vi "Initialize.vi"(7 "Path":path, 8 "error in (no error)":errorcluster, 9 "Invoked from wizard":bool, 10 "Object":T2, 11 "AB_UI_Fmwrk_Build in":refnum<class "AB_UI_Frmwk_Build.lvclass">) -> (0 "error out":errorcluster, 1 "helpTopics out":string[](array[string]), 2 "pageTitles out":string[](array[string]), 3 "AB_UI_Fmwrk_Build out":refnum<class "AB_UI_Frmwk_Build.lvclass">, 4 "helpFile":string, 5 "pageMsgData":T1[](array[typedef]))   [LabVIEW 2020, in "AB_UI_Frmwk_Build.lvclass"]
uses:
  <vilib>/AppBuilder/AB_Classes/Build/UI/AB_UI_Frmwk_Build.lvclass
  <resource>/Framework/Providers/API/ItemRef.ctl
  <resource>/Framework/Providers/Builds/AppBuilder/AB_UI_Page_MessageData.ctl
  <resource>/Framework/Providers/Builds/AppBuilder/AB_UI_Framework_MsgToPage_Action.ctl
  <resource>/Framework/Providers/Builds/AppBuilder/SRdB/AB_SRdB_Action.ctl
  <vilib>/AppBuilder/AB_Classes/Build/AB_Build.lvclass
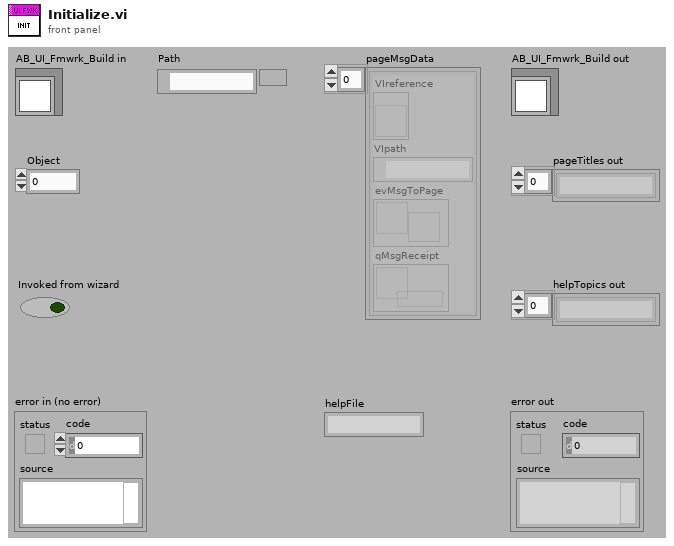
[diagram p1: front panel]
types:
  T1 = typedef "AB_UI_Page_MessageData.ctl" = cluster{"VIreference":refnum<vi>, "VIpath":path, "evMsgToPage":refnum<user-event>, "qMsgReceipt":refnum<queue>}
  T2 = typedef "ItemRef.ctl" = u64
  T3 = typedef "AB_SRdB_Action.ctl" = enum16{"read", "write", "create", "delete", "initialize", "unInitialize", "getLock", "readAll", "writeAll"}
  T4 = typedef "AB_Build.ctl" = cluster{"buildSpecName":string, "buildSpecDescription":string, "destinations":refnum<class "AB_Destination.lvclass">[], "exclusionOption":T5, "defaultLanguage":string, "supportedLanguages":string[], "excludedDirectories":path[], "buildContext":refnum<vi>, "buildObject":T2, "preview":bool, "programatic":bool, "progressBarEvents":T6, "userLog_Path":path, "preActionID":string, "preAction_Path":path, "postActionID":string, "postAction_Path":path, "eng_checkForBrokenVIs?":bool, "eng_verboseLinkerErrors?":bool, "localDest_Path":path, "targetDest_Path":path, "removeVIObject":u16, "cache":refnum<class "PreviewCache.lvclass">, "use cache":bool, "previewCache_ID":string, "buildCache_ID":string, "eng_TempLocalDest_Path":path, "eng_collectDependencies?":bool, "versionInfo":cluster{"buildVersion":cluster{"major":u16, "minor":u16, "patch":u16, "build":u16}, "autoIncrement":bool}, "eng_enableVIChecksums":bool}
  T5 = typedef "AB_Exclusion_Option.ctl" = cluster{"typedefs":bool, "polymorphicVIs":bool, "unusedLibraryItems":bool, "modifyLibraryFile":bool, "edit-timeDependencies":bool, "inlineVIs":bool, "dependent PPLs":bool, "dependent DLLs":bool}
  T6 = typedef "provcom_ProgressBar_Events.ctl" = cluster{"newJob":refnum<user-event>, "newItem":refnum<user-event>, "errorMsg":T7, "cancel":refnum<user-event>}
  T7 = typedef "mxLvBuildError.ctl" = refnum<user-event>
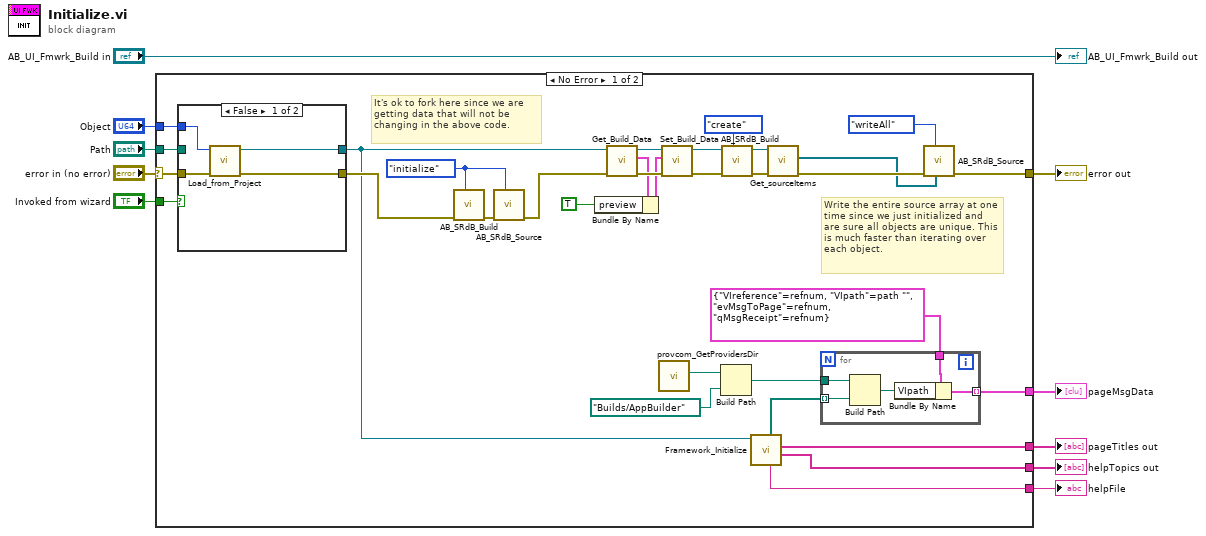
[diagram p0: block diagram]
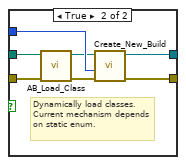
[diagram p2: hidden frame]
diagram:
  n1 = case shown="No Error" "error in (no error)" {
    selector: "error in (no error)" -> [w40 w59]
    tunnel: "Object" -> [w38 _]
    tunnel: [w12 w59] -> w4
    tunnel: [w39 _] -> w5
    tunnel: "Invoked from wizard" -> [w37 _]
    tunnel: [w18 _] -> w1
    tunnel: [w17 _] -> w3
    tunnel: [w19 _] -> w2
    tunnel: "Path" -> [w16 _]
    frame No Error {
      w33 = AB_SRdB_Action."initialize" ("action")
      # "Write the entire source array at one time since we just initialized and are sure all objects are unique. This is much faster than iterating over each object."
      # "It's ok to fork here since we are getting data that will not be changing in the above code."
      n2 = case shown="False" w37 {
        tunnel: [w43 w53] -> w35
        tunnel: w40 -> [w46 w50]
        tunnel: w38 -> [w45 w51]
        tunnel: [w44 w52] -> w21
        tunnel: w16 -> [_ w47]
        frame False {
          n3 = call <vilib>:"Load_from_Project.vi"("error in (no error)"=w46, "Object"=w45) -> ("error out"=w43:errorcluster, "Build out"=w44:refnum<class "AB_Build.lvclass">)  [unwired: 8 out]
        }
        frame True {
          # "Dynamically load classes. Current mechanism depends on static enum."
          n4 = call <vilib>:"AB_Load_Class.vi"("error in (no error)"=w50, "AB_Class path"=w47) -> ("error out"=w49:errorcluster, "AB_Build out"=w48:refnum<class "AB_Build.lvclass">)  [unwired: 8 out]
          n5 = call-dynamic "Create_New_Build.vi"("error in (no error)"=w49, "buildObject"=w51, "AB_Build in"=w48) -> ("error out"=w53:errorcluster, "AB_Build out"=w52:refnum<class "AB_Build.lvclass">)  [unwired: 3 in, 4 out]
        }
      }
      n6 = call <resource>:"AB_SRdB_Build.vi"("action"=w33, "error in (no error)"=w35) -> ("error out"=w34:errorcluster)  [unwired: 1 in, 8 out]
      n7 = call <resource>:"AB_SRdB_Source.vi"("action"=w33, "error in (no error)"=w34) -> ("error out"=w27:errorcluster)  [unwired: 3 in, 6 out]
      n8 = call <vilib>:"Get_Build_Data.vi"("error in (no error)"=w27, "Class in"=w21) -> ("error out"=w26:errorcluster, "data"=w24:T4, "Class out"=w29:refnum<class "AB_Build.lvclass">)  [unwired: 7 out]
      n9 = Bundle By Name(cluster=w24, "preview"=TRUE) -> (w23:T4)
      n10 = call <resource>:"provcom_GetProvidersDir.vi"() -> ("projProv Dir"=w15:path)  [unwired: 11 out]
      n11 = call <vilib>:"Set_Build_Data.vi"("error in (no error)"=w26, "data"=w23, "Class in"=w29) -> ("error out"=w25:errorcluster, "Class out"=w28:refnum<class "AB_Build.lvclass">)  [unwired: 7 out]
      n12 = Build Path(base path=w15, name or relative path=path "Builds/AppBuilder") -> (appended path=w41:path)
      n13 = call <resource>:"AB_SRdB_Build.vi"("action"=AB_SRdB_Action."create", "error in (no error)"=w25, "data in"=w28) -> ("error out"=w30:errorcluster, "data out"=w31:refnum<class "AB_Build.lvclass">)  [unwired: 7 out]
      n14 = call-dynamic "Framework_Initialize.vi"("AB_Build in"=w21) -> ("helpTopics"=w18:string[], "pageTitles"=w19:string[], "helpFile"=w17:string, "pages"=w20:path[])  [unwired: 1 in, 6 out]
      n15 = call <vilib>:"Get_sourceItems.vi"("error in (no error)"=w30, "Class in"=w31) -> ("error out"=w13:errorcluster, "sourceItems"=w11:refnum<class "AB_Source.lvclass">[])  [unwired: 8 out]
      n16 = for {
        tunnel: w41 -> [w58]
        tunnel: [w54] -> w39 mode=indexing
        tunnel: T1 {"VIreference"=refnum, "VIpath"=path "", "evMsgToPage"=refnum, "qMsgReceipt"=refnum} ("qPageMsgs") -> [w56]
        tunnel: w20 -> [w57] mode=indexing
        n17 = Build Path(base path=w58, name or relative path=w57) -> (appended path=w55:path)
        n18 = Bundle By Name(cluster=w56, "VIpath"=w55) -> (w54:T1)
      }
      n19 = call <resource>:"AB_SRdB_Source.vi"("ALL data in"=w11, "action"=AB_SRdB_Action."writeAll", "error in (no error)"=w13) -> ("error out"=w12:errorcluster)  [unwired: 2 in, 6 out]
    }
    frame Error {
    }
  }
  "error out" <- w4
  "pageMsgData" <- w5
  "pageTitles out" <- w2
  "helpTopics out" <- w1
  "helpFile" <- w3
  "AB_UI_Fmwrk_Build out" <- "AB_UI_Fmwrk_Build in"
